vi "Set Window Closeable State.vi"(8 "error in (no error)":errorcluster, 10 "Closeable?":bool) -> (0 "error out":errorcluster)   [LabVIEW 2020, in "UI Manager.lvlib"]
doc: "Sets the closeable state of the window. Setting <b>Closeable?</b> to true enables the close button in the title bar, while setting it to false disables it.\n____\nHAMPEL SOFTWARE ENGINEERING v2.6.0 (2023-12-19 10:54)"
uses:
  UI Manager.lvlib
  Set Window Closeable State Argument--cluster.ctl
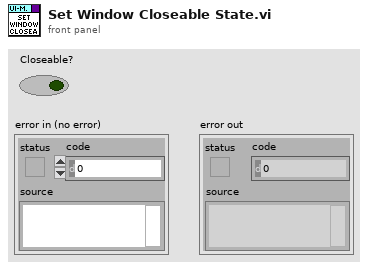
[diagram p1: front panel]
types:
  T1 = typedef "UI Manager.lvlib/Set Window Closeable State Argument--cluster.ctl" = cluster{"Closeable?":bool}
  T2 = typedef "UI Manager.lvlib/Request Events--cluster.ctl" = cluster{"Stop Module":refnum<user-event>, "Show Panel":refnum<user-event>, "Hide Panel":refnum<user-event>, "Get Module Execution Status":refnum<user-event>, "Show Diagram":refnum<user-event>, "Set Run-Time Menu":refnum<user-event>, "Show HSE-ABOUT":refnum<user-event>, "Show PROJECT-ABOUT":refnum<user-event>, "Configure":refnum<user-event>, "Prepare":refnum<user-event>, "Update Status Bar":refnum<user-event>, "Trigger System Message":refnum<user-event>, "Add Module to Run-Time Menu":refnum<user-event>, "Set Modules":refnum<user-event>, "Register for Module Events":refnum<user-event>, "Display another Module UI":refnum<user-event>, "Set Run-Time Menu Visibility":refnum<user-event>, "Set Window Closeable State":refnum<user-event>, "Shutdown Application":refnum<user-event>, "Remove Module from Run-Time Menu":refnum<user-event>, "Set CLI Arguments":refnum<user-event>, "Get CLI Arguments":refnum<user-event>, "External Login":refnum<user-event>, "Get User Level":refnum<user-event>}
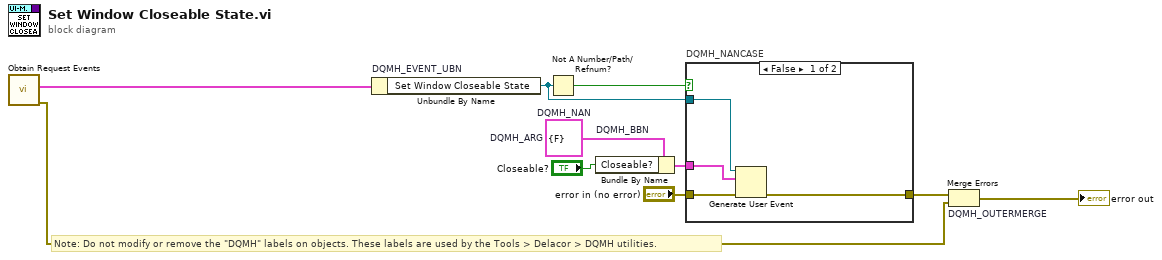
[diagram p0: block diagram]
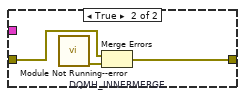
[diagram p2: hidden frame]
diagram:
  w4 = T1 {"Closeable?"=FALSE}  # DQMH_ARG
  # "Note: Do not modify or remove the \"DQMH\" labels on objects. These labels are used by the Tools > Delacor > DQMH utilities."
  n1 = call "Obtain Request Events.vi"() -> ("error out"=w2:errorcluster, "UI Manager Request Events"=w1:T2)  [unwired: 10 in]
  n2 = Unbundle By Name "DQMH_EVENT_UBN"(w1) -> ("Set Window Closeable State"=w6:refnum<user-event>)
  n3 = Not A Number/Path/Refnum? "DQMH_NAN"(number/path/refnum=w6) -> (NaN/Path/Refnum?=w7:bool)
  n4 = Bundle By Name "DQMH_BBN"(cluster=w4, "Closeable?"="Closeable?") -> (w8:T1)
  n5 = case "DQMH_NANCASE" shown="False" w7 {
    tunnel: "error in (no error)" -> [w14 w17]
    tunnel: [w13 w16] -> w5
    tunnel: w6 -> [w12 _]
    tunnel: w8 -> [w11 _]
    frame False {
      n6 = Generate User Event(user event=w12, event data cluster=w11, error in=w14) -> (error out=w13:errorcluster)  [unwired: 1 in, 1 out]
    }
    frame True {
      n7 = call "Module Not Running--error.vi"() -> ("error out"=w15:errorcluster)  [unwired: 11 in]
      n8 = Merge Errors "DQMH_INNERMERGE"(w17, w15) -> (w16:errorcluster)
    }
  }
  n9 = Merge Errors "DQMH_OUTERMERGE"(w5, w2) -> (→"error out":errorcluster)
